vi "CalculateCheckSum.vi"(11 "strInput":string) -> (3 "strOut":string)   [LabVIEW 2011]
panel:
  out "路径":path
  out "Path":string
  out "strArrayBuf":string[](array[string])
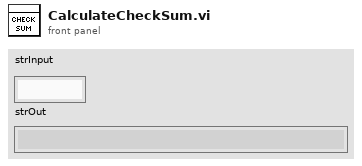
[diagram p1: front panel]
types:
  T1 = enum16{"open", "replace", "create", "open or create", "replace or create", "replace or create with confirmation"}
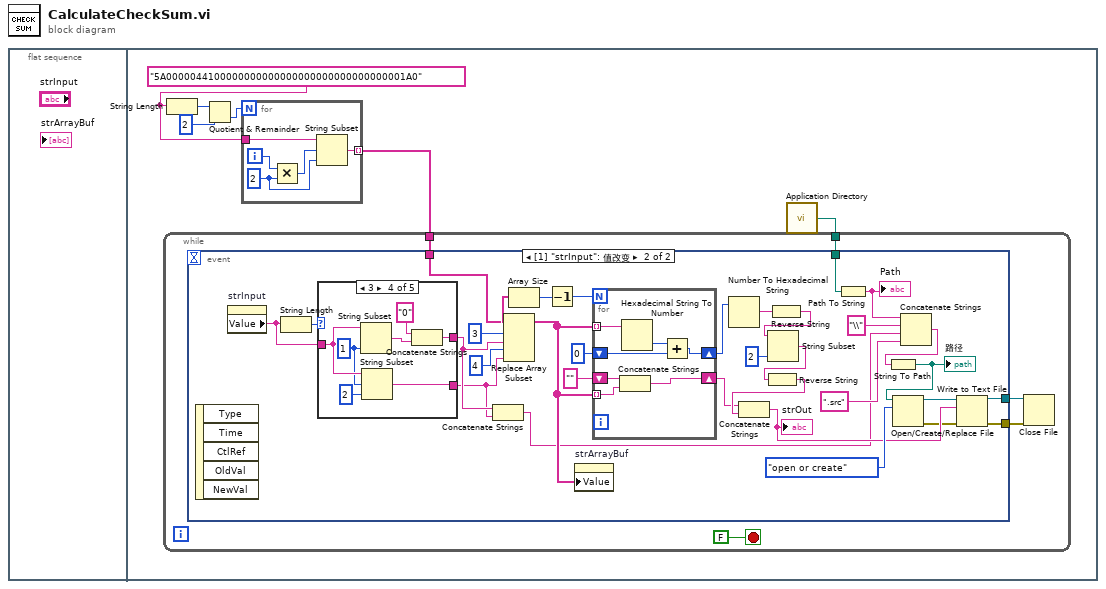
[diagram p0: block diagram]
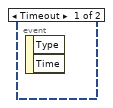
[diagram p2: hidden frame]
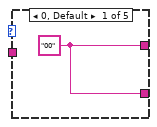
[diagram p3: hidden frame]
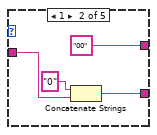
[diagram p4: hidden frame]
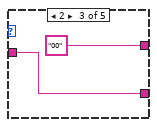
[diagram p5: hidden frame]
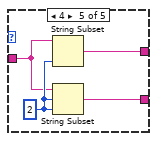
[diagram p6: hidden frame]
diagram:
  n1 = flat-sequence {
    frame #0 {
    }
    frame #1 {
      w6 = "5A0000044100000000000000000000000000000001A0"
      n2 = String Length(string=w6) -> (length=w4:i32)
      n3 = Quotient & Remainder(x=w4, y=2) -> (floor(x/y)=w5:i32)  [unwired: 1 out]
      n4 = for {
        N: w5 -> [_]
        tunnel: w6 -> [w73]
        tunnel: [w69] -> w2 mode=indexing
        i -> [w70]
        w71 = 2 ("y")
        n5 = Multiply(x=w70, y=w71) -> (x*y=w72:i32)
        n6 = String Subset(string=w73, offset (0)=w72, length (rest)=w71) -> (substring=w69:string)
      }
      n7 = call <vilib>:"Application Directory.vi"() -> ("Application Directory"=w1:path)
      n8 = while {
        tunnel: w2 -> [w10]
        tunnel: w1 -> [w9]
        stop <- FALSE stop-if-true
        n9 = event shown="[1] \"strInput\": 值改变" {
          selector: _ -> [_ _]
          dyn-events: _ -> [_ _]
          timeout: _ -> [_ _]
          tunnel: w10 -> [_ w27]
          tunnel: w9 -> [_ w26]
          tunnel: [_ w16] -> w8
          tunnel: [_ w15] -> w7
          event Timeout {
            n10 = event-data() -> ()  [unwired: 1 in, 2 out]
          }
          event "strInput": Value Change {
            n11 = event-data() -> ()  [unwired: 1 in, 5 out]
            n12 = property on="strInput" class="Str"() -> ("Value"=w28:string)  [unwired: 2 in, 2 out]
            n13 = String Length(string=w28) -> (length=w29:i32)
            n14 = case shown="3" w29 {
              tunnel: w28 -> [_ w52 w56 w64 w67]
              tunnel: [w51 "00" "00" w58 w66] -> w14
              tunnel: [w51 w54 w56 w61 w65] -> w13
              frame 0, Default {
                w51 = "00"
              }
              frame 1 {
                n15 = Concatenate Strings("0", w52) -> (w54:string)
              }
              frame 2 {
              }
              frame 3 {
                w63 = 1 ("长度（剩余）")
                n16 = String Subset(string=w64, length (rest)=w63) -> (substring=w59:string)  [unwired: 1 in]
                n17 = String Subset(string=w64, offset (0)=w63, length (rest)=2 ("长度（剩余）")) -> (substring=w61:string)
                n18 = Concatenate Strings("0", w59) -> (w58:string)
              }
              frame 4 {
                w68 = 2 ("偏移量(0)")
                n19 = String Subset(string=w67, length (rest)=w68) -> (substring=w66:string)  [unwired: 1 in]
                n20 = String Subset(string=w67, offset (0)=w68, length (rest)=w68) -> (substring=w65:string)
              }
            }
            n21 = Concatenate Strings(w14, w13) -> (w12:string)
            n22 = Replace Array Subset(array=w27, new element #1=w14, index #1=3 ("索引"), new element #2=w13, index #2=4 ("索引")) -> (w41:string[])
            n23 = Array Size(array=w41) -> (size(s)=w32:i32)
            n24 = Decrement(x=w32) -> (x-1=w33:i32)
            n25 = property on="strArrayBuf" class="Arr (严格)"("Value"=w41) -> ()  [unwired: 2 in, 2 out]
            n26 = for {
              N: w33 -> [_]
              tunnel: w41 -> [w50] mode=indexing
              shift-right: [w47] -> w35
              shift-left: 0 -> [w48]
              shift-right: [w46] -> w42
              shift-left: "" -> [w45]
              tunnel: w41 -> [w44] mode=indexing
              n27 = Concatenate Strings(w45, w44) -> (w46:string)
              n28 = Hexadecimal String To Number(string=w50) -> (number=w49:u32)  [unwired: 2 in, 1 out]
              n29 = Add(x=w49, y=w48) -> (x+y=w47:u32)
            }
            n30 = Number To Hexadecimal String(2:w35) -> (0:w36:string)  [unwired: 1 in]
            n31 = Reverse String(1:w36) -> (0:w37:string)
            n32 = String Subset(string=w37, length (rest)=2 ("长度（剩余）")) -> (substring=w39:string)  [unwired: 1 in]
            n33 = Reverse String(1:w39) -> (0:w43:string)
            n34 = Concatenate Strings(w42, w43) -> (w18:string)
            "strOut" <- w18
            n35 = Path To String(path=w26) -> (string=w25:string)
            "Path" <- w25
            n36 = Concatenate Strings(w25, "\\" ("字符串"), w12, ".src" ("字符串")) -> (w23:string)
            n37 = String To Path(string=w23) -> (path=w21:path)
            "路径" <- w21
            n38 = Open/Create/Replace File(file path (use dialog)=w21, operation (0:open)=T1."open or create" ("操作(0:open)")) -> (refnum out=w19:refnum<file>, error out=w17:errorcluster)  [unwired: 4 in, 1 out]
            n39 = Write to Text File(file (use dialog)=w19, text=w18, error in=w17) -> (refnum out=w16:refnum<file>, error out=w15:errorcluster)  [unwired: 1 in, 1 out]
          }
        }
        n40 = Close File(refnum=w8, error in=w7) -> ()  [unwired: 2 out]
      }
    }
  }
